vi "perteneceAtorre.vi"(0 "P1":cluster{"x":dbl, "y":dbl}, 1 "P2":cluster{"x":dbl, "y":dbl}, 2 "P":cluster{"x":dbl, "y":dbl}, 3 "P3":cluster{"x":dbl, "y":dbl}, 4 "P4":cluster{"x":dbl, "y":dbl}) -> (5 "out":bool)   [LabVIEW 2020]
panel:
  # "Coordenadas del Rectangulo"
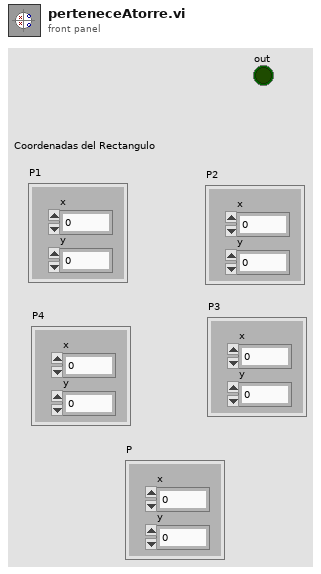
[diagram p1: front panel]
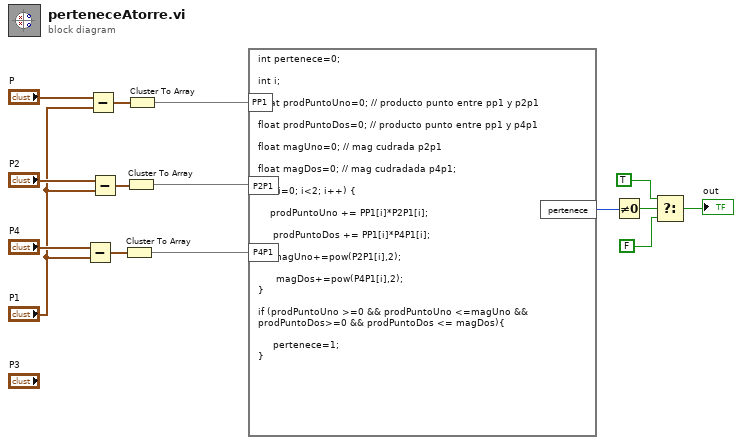
[diagram p0: block diagram]
diagram:
  n1 = Subtract(x="P4", y="P1") -> (x-y=w9:cluster{"x":dbl, "y":dbl})
  n2 = Subtract(x="P", y="P1") -> (x-y=w11:cluster{"x":dbl, "y":dbl})
  n3 = Subtract(x="P2", y="P1") -> (x-y=w10:cluster{"x":dbl, "y":dbl})
  n4 = Cluster To Array(cluster=w9) -> (array=w6:dbl[])
  n5 = Cluster To Array(cluster=w10) -> (array=w7:dbl[])
  n6 = Cluster To Array(cluster=w11) -> (array=w8:dbl[])
  n7 = formula code="int pertenece=0;\n\nint i;\n \nfloat prodPuntoUno=0; // producto punto entre pp1 y p2p1\n\nfloat prodPuntoDos=0; // producto punto entre pp1 y p4p1\n\nfloat magUno=0; // mag cudrada p2p1\n\nfloat magDos=0; // mag cudradada p4p1;\n\nfor (i=0; i<2; i++) {\n\n    prodPuntoUno += PP1[i]*P2P1[i];\n\n     prodPuntoDos += PP1[i]*P4P1[i];\n\n     magUno+=pow(P2P1[i],2);\n\n      magDos+=pow(P4P1[i],2);\n}\n\nif (prodPuntoUno >=0 && prodPuntoUno <=magUno && prodPuntoDos>=0 && prodPuntoDos <= magDos){\n\n     pertenece=1;\n}"("PP1"=w8, "P2P1"=w7, "P4P1"=w6) -> ("pertenece"=w5:i32)
  n8 = Not Equal To 0?(x=w5) -> (x != 0?=w4:bool)
  n9 = Select(t=TRUE, s=w4, f=FALSE) -> (s? t:f=→"out":bool)
